vi "Get Array Element TD.vi"(8 "错误输入":errorcluster, 10 "Array":variant) -> (0 "错误输出":errorcluster, 2 "Type Descriptor":T1)   [LabVIEW 2012, in "TD Tools.lvlib"]
uses:
  TD Tools.lvlib
  Custom Type/Type Descriptor.ctl
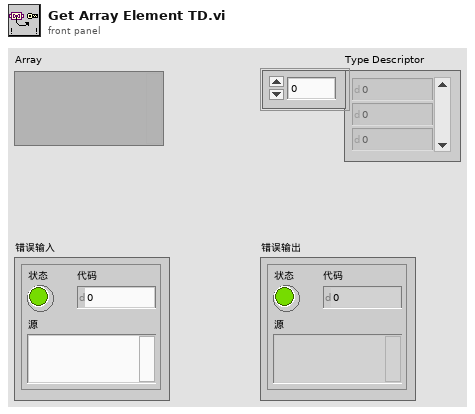
[diagram p1: front panel]
types:
  T1 = typedef "TD Tools.lvlib/Type Descriptor.ctl" = u16[]
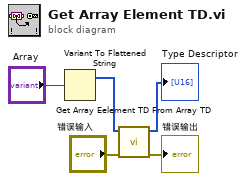
[diagram p0: block diagram]
diagram:
  n1 = Variant To Flattened String(Variant="Array") -> (1:w4:i16[])  [unwired: 1 out]
  n2 = call "Get Array Eelement TD From Array TD.vi"("错误输入"="错误输入", "Array Type Descriptor"=w4) -> ("错误输出"=→"错误输出":errorcluster, "Element Type Descriptor"=→"Type Descriptor":T1)  [unwired: 8 in]
